vi "Broadcast Connected Clients.vi"(8 "error in (no error)":errorcluster, 11 "Websocket Server in":refnum<class "WS Server.lvclass">) -> (0 "error out":errorcluster, 3 "Websocket Server out":refnum<class "WS Server.lvclass">)   [LabVIEW 2016, in "WebSocket Networking.lvlib" / "WS Server.lvclass"]
uses:
  <userlib>/Common Components/WebSocket Networking/WS Server/WS Server.lvclass
  <userlib>/Common Components/WebSocket Networking/Message 2D String Array/Message 2D String Array.lvclass
  C:/Program Files (x86)/National Instruments/LabVIEW 2016/user.lib/Composed Systems/Stream/Mediator/Classes/Message Interface/Message Interface.lvclass
  <userlib>/Common Components/WebSocket Networking/WS Server/WS Server.lvclass/WS Server.ctl
  <userlib>/Composed Systems/Stream/Mediator/Classes/Message Transport Queue/Message Transport Queue.lvclass
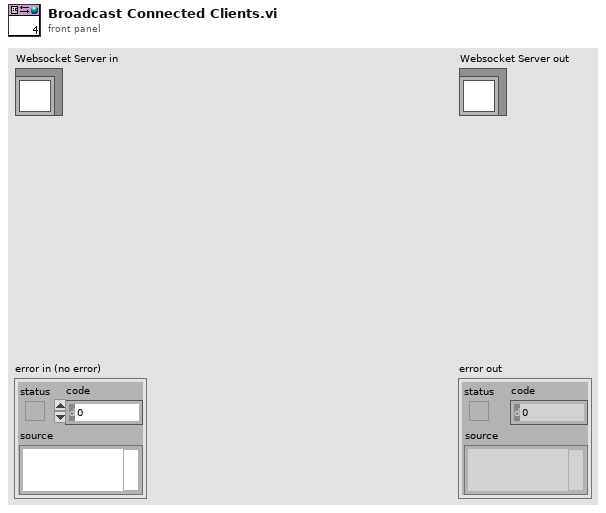
[diagram p1: front panel]
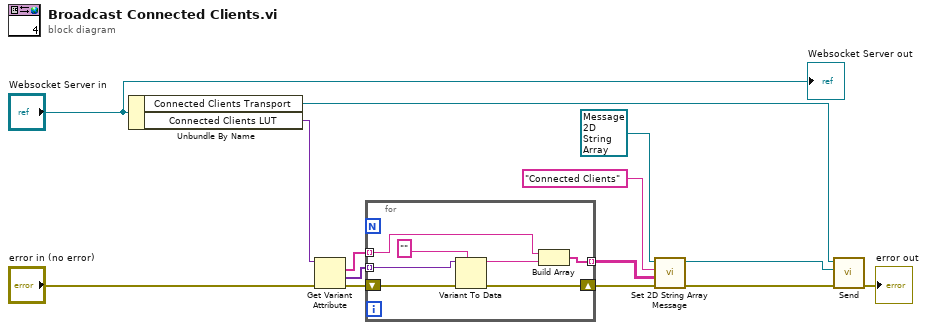
[diagram p0: block diagram]
diagram:
  n1 = Unbundle By Name("Websocket Server in") -> ("Connected Clients Transport"=w7:refnum<class "Message Transport Queue.lvclass">, "Connected Clients LUT"=w11:variant)
  n2 = Get Variant Attribute(Variant=w11, error in="error in (no error)") -> (names=w1:string[], values=w10:variant[], error out=w5:errorcluster)  [unwired: 2 in, 1 out]
  n3 = for {
    tunnel: w10 -> [w21] mode=indexing
    tunnel: [w18] -> w9 mode=indexing
    shift-right: [w19] -> w4
    shift-left: w5 -> [w20]
    tunnel: w1 -> [w17] mode=indexing
    n4 = Variant To Data(error in=w20, type="", Variant=w21) -> (data=w15:string, error out=w19:errorcluster)
    n5 = Build Array(w17, w15) -> (w18:string[])
  }
  n6 = call <userlib>:"Set 2D String Array Message.vi"("error in (no error)"=w4, "Value"=w9, "Name"="Connected Clients", "Message Double in"=refnum<class "Message 2D String Array.lvclass"> refnum ("Stream Mediator.lvlib:Message 2D String Array.lvclass")) -> ("error out"=w3:errorcluster, "Message Double out"=w8:refnum<class "Message 2D String Array.lvclass">)  [unwired: 6 in]
  n7 = call-dynamic "Send.vi"("error in (no error)"=w3, "Message"=w8, "Message Transport Queue in"=w7) -> ("error out"=→"error out":errorcluster)  [unwired: 6 in, 2 out]
  "Websocket Server out" <- "Websocket Server in"
